vi "GET_PRESTATUS.vi"(10 "CODE_ID":string, 11 "PRODUCT_ID":string) -> (3 "OK?":bool)   [LabVIEW 2020]
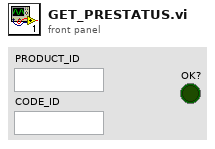
[diagram p1: front panel]
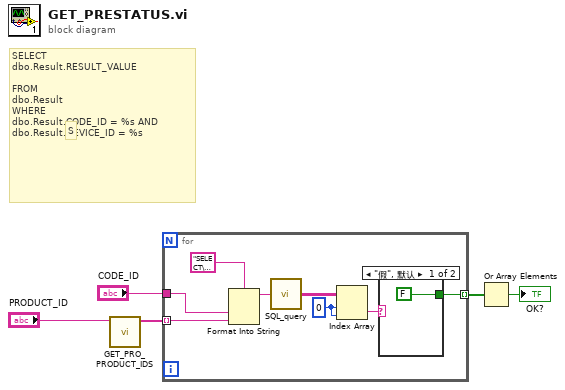
[diagram p0: block diagram]
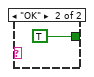
[diagram p2: hidden frame]
diagram:
  # "SELECT\ndbo.Result.RESULT_VALUE\n\nFROM\ndbo.Result\nWHERE\ndbo.Result.CODE_ID = %s AND\ndbo.Result.DEVICE_ID = %s"
  # "S"
  n1 = call "GET_PRO_PRODUCT_IDS.vi"("PRODUCT_ID"="PRODUCT_ID") -> ("前序工位"=w4:string[])  [unwired: 10 in]
  n2 = for {
    tunnel: w4 -> [w12] mode=indexing
    tunnel: "CODE_ID" -> [w11]
    tunnel: [w6] -> w2 mode=indexing
    w7 = 0 ("索引 (行)")
    n3 = Format Into String(format string="SELECT\ndbo.Result.RESULT_VALUE\n\nFROM\ndbo.Result\nWHERE\ndbo.Result.CODE_ID = %s AND\ndbo.Result.DEVICE_ID = %s\n" ("格式字符串"), w11, w12) -> (resulting string=w10:string)  [unwired: 2 in, 1 out]
    n4 = call "SQL_query.vi"("SQL query"=w10) -> ("data"=w9:string[][])  [unwired: 3 in, 1 out]
    n5 = Index Array(array=w9, index (row)=w7, index (col)=w7) -> (element=w8:string)
    n6 = case shown="\"假\", 默认" w8 {
      tunnel: [FALSE TRUE] -> w6
      frame "假", Default {
      }
      frame "OK" {
      }
    }
  }
  n7 = Or Array Elements(Boolean array=w2) -> (logical OR=→"OK?":bool)
